vi "JSON_Application_Parser (SubVI).vi"(6 "data":string, 8 "error in (no error)":errorcluster, 9 "RequestNumber":i32, 10 "ID":i32) -> (0 "error out":errorcluster, 2 "Cluster":T1)   [LabVIEW 2018]
uses:
  <vilib>/addons/database/Auxilliary.llb/DB Tools Column Info.ctl
  <vilib>/addons/database/Auxilliary.llb/DB Tools DataTypes.ctl
  <vilib>/addons/database/NI_Database_API.lvlib
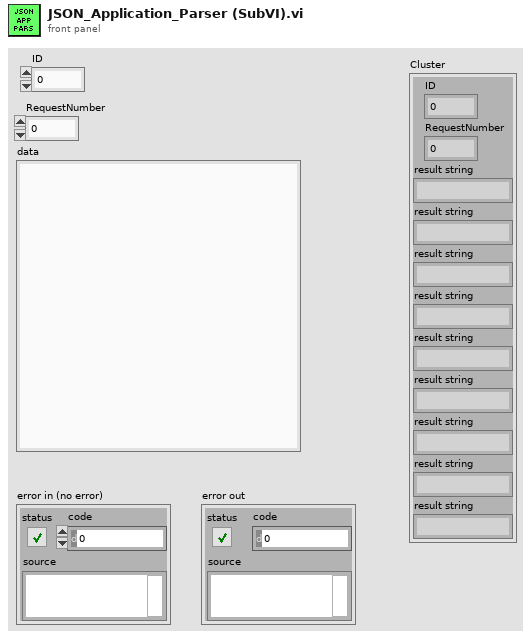
[diagram p1: front panel]
types:
  T1 = cluster{"ID":i32, "RequestNumber":i32, "result string":string, "result string":string, "result string":string, "result string":string, "result string":string, "result string":string, "result string":string, "result string":string, "result string":string}
  T2 = typedef "NI_Database_API.lvlib/DB Tools Column Info.ctl" = cluster{"column name":string, "data type":T3, "size":i32, "allow null?":bool}
  T3 = typedef "NI_Database_API.lvlib/DB Tools DataTypes.ctl" = enum16{"String", "Long (I32)", "Single (SGL)", "Double (DBL)", "Date/Time", "Binary"}
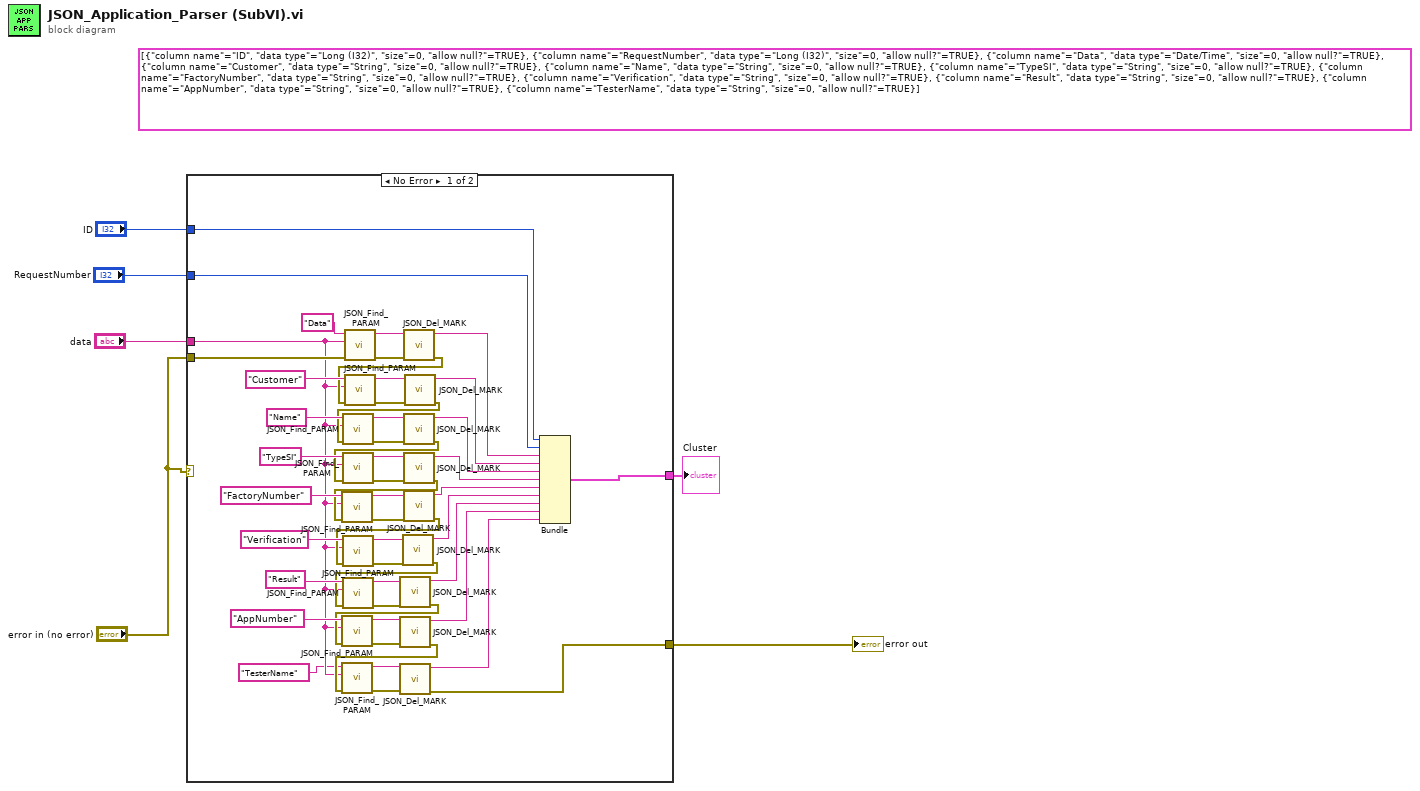
[diagram p0: block diagram]
diagram:
  (unwired) T2[] [{"column name"="ID", "data type"=enum."Long (I32)", "size"=0, "allow null?"=TRUE}, {"column name"="RequestNumber", "data type"=enum."Long (I32)", "size"=0, "allow null?"=TRUE}, {"column name"="Data", "data type"=enum."Date/Time", "size"=0, "allow null?"=TRUE}, {"column name"="Customer", "data type"=enum."String", "size"=0, "allow null?"=TRUE}, {"column name"="Name", "data type"=enum."String", "size"=0, "allow null?"=TRUE}, {"column name"="TypeSI", "data type"=enum."String", "size"=0, "allow null?"=TRUE}, {"column name"="FactoryNumber", "data type"=enum."String", "size"=0, "allow null?"=TRUE}, {"column name"="Verification", "data type"=enum."String", "size"=0, "allow null?"=TRUE}, {"column name"="Result", "data type"=enum."String", "size"=0, "allow null?"=TRUE}, {"column name"="AppNumber", "data type"=enum."String", "size"=0, "allow null?"=TRUE}, {"column name"="TesterName", "data type"=enum."String", "size"=0, "allow null?"=TRUE}] ("column information")
  n1 = case shown="No Error" "error in (no error)" {
    tunnel: [w10 w57] -> w6
    tunnel: "error in (no error)" -> [w56 w57]
    tunnel: "data" -> [w8 _]
    tunnel: "RequestNumber" -> [w15 _]
    tunnel: [w23 _] -> w1
    tunnel: "ID" -> [w14 _]
    frame No Error {
      n2 = call "JSON_Find_PARAM.vi"("error in (no error)"=w56, "data"=w8, "name"="Data") -> ("error out"=w32:errorcluster, "String"=w33:string)  [unwired: 7 in]
      n3 = call "JSON_Del_MARK.vi"("error in (no error)"=w32, "String"=w33) -> ("error out"=w22:errorcluster, "result string"=w48:string)  [unwired: 8 in]
      n4 = call "JSON_Find_PARAM.vi"("error in (no error)"=w22, "data"=w8, "name"="Customer") -> ("error out"=w35:errorcluster, "String"=w34:string)  [unwired: 7 in]
      n5 = call "JSON_Del_MARK.vi"("error in (no error)"=w35, "String"=w34) -> ("error out"=w21:errorcluster, "result string"=w49:string)  [unwired: 8 in]
      n6 = call "JSON_Find_PARAM.vi"("error in (no error)"=w21, "data"=w8, "name"="Name") -> ("error out"=w37:errorcluster, "String"=w36:string)  [unwired: 7 in]
      n7 = call "JSON_Del_MARK.vi"("error in (no error)"=w37, "String"=w36) -> ("error out"=w20:errorcluster, "result string"=w50:string)  [unwired: 8 in]
      n8 = call "JSON_Find_PARAM.vi"("error in (no error)"=w20, "data"=w8, "name"="TypeSI") -> ("error out"=w39:errorcluster, "String"=w38:string)  [unwired: 7 in]
      n9 = call "JSON_Del_MARK.vi"("error in (no error)"=w39, "String"=w38) -> ("error out"=w19:errorcluster, "result string"=w51:string)  [unwired: 8 in]
      n10 = call "JSON_Find_PARAM.vi"("error in (no error)"=w19, "data"=w8, "name"="FactoryNumber") -> ("error out"=w41:errorcluster, "String"=w40:string)  [unwired: 7 in]
      n11 = call "JSON_Del_MARK.vi"("error in (no error)"=w41, "String"=w40) -> ("error out"=w18:errorcluster, "result string"=w52:string)  [unwired: 8 in]
      n12 = call "JSON_Find_PARAM.vi"("error in (no error)"=w18, "data"=w8, "name"="Verification") -> ("error out"=w43:errorcluster, "String"=w42:string)  [unwired: 7 in]
      n13 = call "JSON_Del_MARK.vi"("error in (no error)"=w43, "String"=w42) -> ("error out"=w17:errorcluster, "result string"=w53:string)  [unwired: 8 in]
      n14 = call "JSON_Find_PARAM.vi"("error in (no error)"=w17, "data"=w8, "name"="Result") -> ("error out"=w45:errorcluster, "String"=w44:string)  [unwired: 7 in]
      n15 = call "JSON_Del_MARK.vi"("error in (no error)"=w45, "String"=w44) -> ("error out"=w16:errorcluster, "result string"=w54:string)  [unwired: 8 in]
      n16 = call "JSON_Find_PARAM.vi"("error in (no error)"=w16, "data"=w8, "name"="AppNumber") -> ("error out"=w47:errorcluster, "String"=w46:string)  [unwired: 7 in]
      n17 = call "JSON_Del_MARK.vi"("error in (no error)"=w47, "String"=w46) -> ("error out"=w11:errorcluster, "result string"=w55:string)  [unwired: 8 in]
      n18 = call "JSON_Find_PARAM.vi"("error in (no error)"=w11, "data"=w8, "name"="TesterName") -> ("error out"=w13:errorcluster, "String"=w12:string)  [unwired: 7 in]
      n19 = call "JSON_Del_MARK.vi"("error in (no error)"=w13, "String"=w12) -> ("error out"=w10:errorcluster, "result string"=w9:string)  [unwired: 8 in]
      n20 = Bundle("ID"=w14, "RequestNumber"=w15, "result string"=w48, "result string"=w49, "result string"=w50, "result string"=w51, "result string"=w52, "result string"=w53, "result string"=w54, "result string"=w55, "result string"=w9) -> (w23:T1)  [unwired: 1 in]
    }
    frame Error {
    }
  }
  "error out" <- w6
  "Cluster" <- w1
